vi "Gestione tabella ricerca collaudi.vi"() -> ()   [LabVIEW 2019]
uses:
  Global percorso impostazioni.vi
  <vilib>/Utility/file.llb/Read Delimited Spreadsheet (string).vi
  <vilib>/Utility/file.llb/Write Delimited Spreadsheet (string).vi
  <vilib>/addons/database/NI_Database_API.lvlib
panel:
  in  "aggiungi tutti":bool
  in  "aggiungi":bool
  in  "salva":bool
  out "String":string
  in  "rimuovi selezionata tri":bool
  in  "Lista colonne da visualizzare":i32(listbox)
  in  "exit":bool
  in  "Lista colonne":i32(listbox)
  # "GESTIONE TABELLA RICERCA COLLAUDI"
  # "Nota: trascina per ordinare"
  # "Nota: trascina per ordinare"
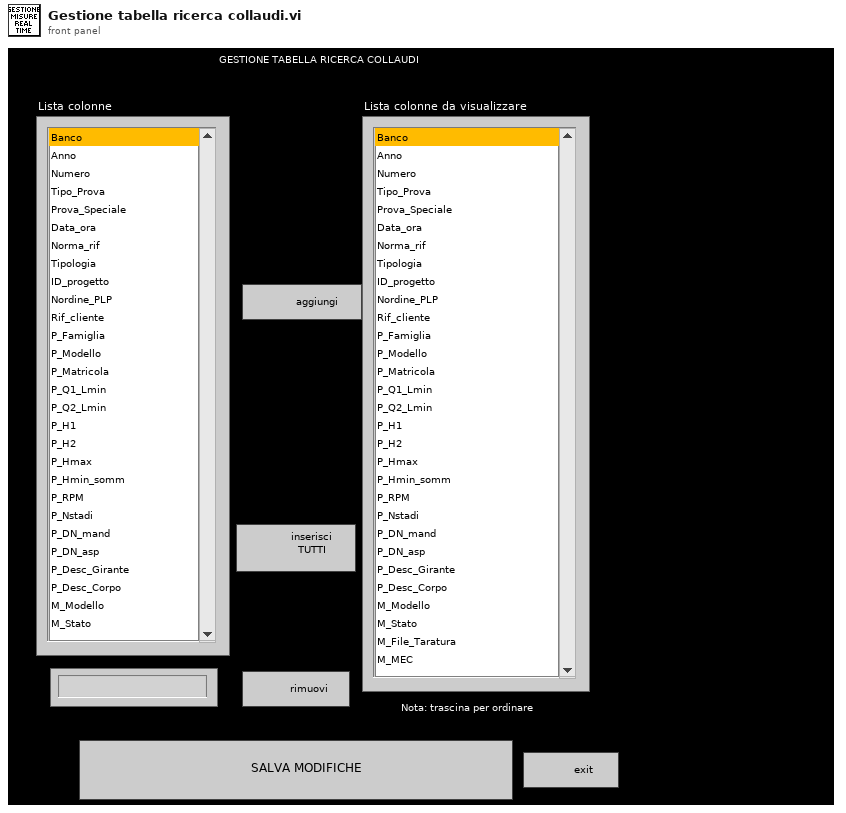
[diagram p1: front panel]
types:
  T1 = typedef "NI_Database_API.lvlib/Conn ObjectReference.ctl" = refnum<k1>
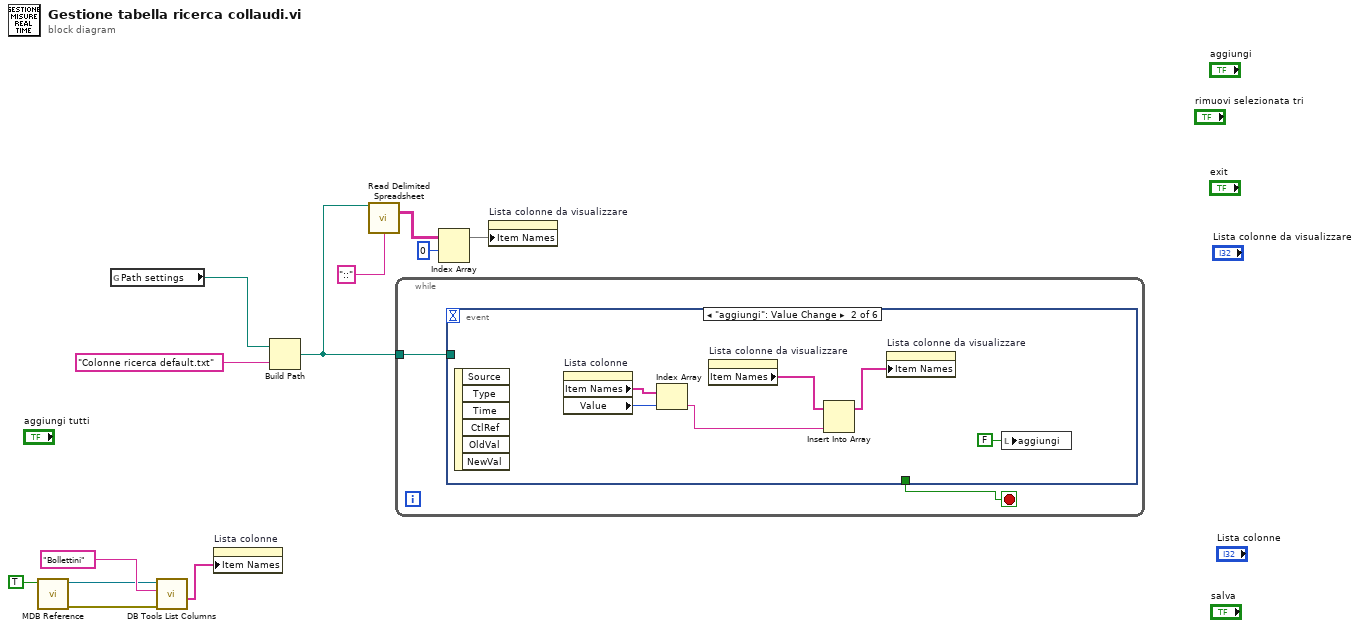
[diagram p0: block diagram]
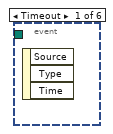
[diagram p2: hidden frame]
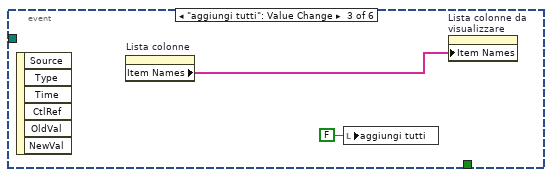
[diagram p3: hidden frame]
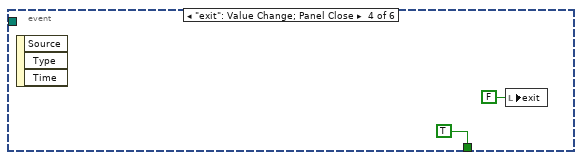
[diagram p4: hidden frame]
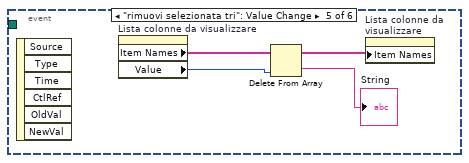
[diagram p5: hidden frame]
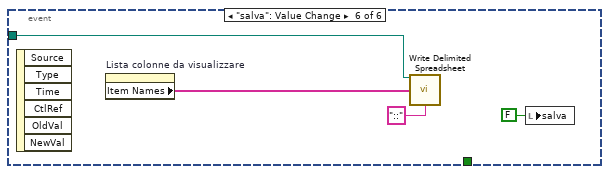
[diagram p6: hidden frame]
diagram:
  n1 = call "MDB Reference.vi"("Collaudi T/motori F"=TRUE ("NM?")) -> ("error out"=w9:errorcluster, "Refnum out"=w10:T1)  [unwired: 8 in, 1 out]
  n2 = global read "Global percorso impostazioni.vi" "Path settings"() -> (w1:path)
  n3 = call <vilib>:"DB Tools List Columns.vi"("error in (no error)"=w9, "table"="Bollettini", "connection reference"=w10) -> ("columns"=w8:string[])  [unwired: 1 in, 3 out]
  n4 = property on="Lista colonne" class="LstBox (strict)"("Item Names"=w8) -> ()  [unwired: 2 in, 2 out]
  n5 = Build Path(base path=w1, name or relative path="Colonne ricerca default.txt") -> (appended path=w6:path)
  n6 = call-poly <vilib>:"Read Delimited Spreadsheet.vi"("file path (dialog if empty)"=w6, "delimiter (\\t)"="::" ("delimiter (\\t)")) -> ("all rows"=w5:string[][])  [unwired: 8 in, 5 out]
  n7 = while {
    tunnel: w6 -> [w13]
    stop <- w14 stop-if-true
    n8 = event shown="[1] \"aggiungi\": Value Change" {
      selector: _ -> [_ _ _ _ _ _]
      dyn-events: _ -> [_ _ _ _ _ _]
      timeout: _ -> [_ _ _ _ _ _]
      tunnel: [_ _ _ TRUE _ _] -> w14
      tunnel: w13 -> [_ _ _ _ _ w30]
      event Timeout {
        n9 = event-data() -> ()  [unwired: 1 in, 3 out]
      }
      event "aggiungi": Value Change {
        n10 = event-data() -> ()  [unwired: 1 in, 6 out]
        n11 = property on="Lista colonne" class="LstBox (strict)"() -> ("Item Names"=w20:string[], "Value"=w19:i32)  [unwired: 2 in, 2 out]
        n12 = Index Array(array=w20, index=w19) -> (element=w16:string)
        n13 = property on="Lista colonne da visualizzare" class="LstBox (strict)"() -> ("Item Names"=w18:string[])  [unwired: 2 in, 2 out]
        n14 = Insert Into Array(array=w18, new element=w16) -> (w17:string[])  [unwired: 1 in]
        n15 = property on="Lista colonne da visualizzare" class="LstBox (strict)"("Item Names"=w17) -> ()  [unwired: 2 in, 2 out]
        n16 = local write "aggiungi"(FALSE ("aggiungi")) -> ()
      }
      event "aggiungi tutti": Value Change {
        n17 = event-data() -> ()  [unwired: 1 in, 6 out]
        n18 = property on="Lista colonne" class="LstBox (strict)"() -> ("Item Names"=w22:string[])  [unwired: 2 in, 2 out]
        n19 = local write "aggiungi tutti"(FALSE ("aggiungi tutti")) -> ()
        n20 = property on="Lista colonne da visualizzare" class="LstBox (strict)"("Item Names"=w22) -> ()  [unwired: 2 in, 2 out]
      }
      event "exit": Value Change; Panel Close {
        n21 = event-data() -> ()  [unwired: 1 in, 3 out]
        n22 = local write "exit"(FALSE ("exit")) -> ()
      }
      event "rimuovi selezionata tri": Value Change {
        n23 = event-data() -> ()  [unwired: 1 in, 6 out]
        n24 = property on="Lista colonne da visualizzare" class="LstBox (strict)"() -> ("Item Names"=w28:string[], "Value"=w27:i32)  [unwired: 2 in, 2 out]
        n25 = Delete From Array(array=w28, index=w27) -> (deleted portion=→"String":string, array with subset deleted=w26:string[])  [unwired: 1 in]
        n26 = property on="Lista colonne da visualizzare" class="LstBox (strict)"("Item Names"=w26) -> ()  [unwired: 2 in, 2 out]
      }
      event "salva": Value Change {
        n27 = event-data() -> ()  [unwired: 1 in, 6 out]
        n28 = property on="Lista colonne da visualizzare" class="LstBox (strict)"() -> ("Item Names"=w31:string[])  [unwired: 2 in, 2 out]
        n29 = call-poly <vilib>:"Write Delimited Spreadsheet.vi"("file path (dialog if empty)"=w30, "1D data"=w31, "delimiter (\\t)"="::" ("delimiter (\\t)")) -> ()  [unwired: 11 in, 2 out]
        n30 = local write "salva"(FALSE ("salva")) -> ()
      }
    }
  }
  n31 = Index Array(array=w5, index (row)=0) -> (element=w4:string[])  [unwired: 1 in]
  n32 = property on="Lista colonne da visualizzare" class="LstBox (strict)"("Item Names"=w4) -> ()  [unwired: 2 in, 2 out]
